vi "PXI_Host_U16_Write_OldMethod_Benchmark.vi"() -> ()   [LabVIEW 2018]
uses:
  <vilib>/Platform/TimedLoop/XDataNode/timing_clust.ctl
  <vilib>/Platform/TimedLoop/XDataNode/nitl_modes.ctl
  <vilib>/Platform/TimedLoop/XDataNode/wakeup.ctl
  <vilib>/NI/LVFPGA Adv Session Resources/OpenByNameSubVI.vi
  <vilib>/rvi/interface/common/dynamic/niFpgaEscapeDelimiterAndNull.vi
  <vilib>/Utility/error.llb/Error Cluster From Error Code.vi
  <vilib>/rvi/errors/niLvFpgaAdjustHostInterfaceError.vi
  <vilib>/FPGAPlugInAG/Dynamic/niLvFpga_Close_Dynamic.vi
  <vilib>/platform/TimedLoop/XDataNode/XDataNode.xnode
  <vilib>/NI/LVFPGA Adv Session Resources/OpenByName.xnode
  <vilib>/rvi/interface/nirviReadWriteControl/nirviReadWriteControl.xnode
  <vilib>/rvi/interface/nirviCloseFPGA/nirviCloseFPGA.xnode
  NiFpgaLv.dll
  <vilib>/rvi/interface/Simulation/niFpgaSimulationCallBeginRW.vi
  <vilib>/NI/LVFPGA Adv Session Resources/LVFPGAAdvSessionResources.lvlib
  cRIO RT/FPGA Bitfile Register Operations/Scalar IO Operations/FPGA Register IO.lvlib
  <vilib>/Platform/TimedLoop/XDataNode/XDNodeRunTimeDep.lvlib
panel:
  out "Maximum(s)":dbl
  out "Standard deviation":dbl
  out "Waveform Graph":dbl[](graph)
  out "error out":errorcluster
  out "Execution time (s)":dbl
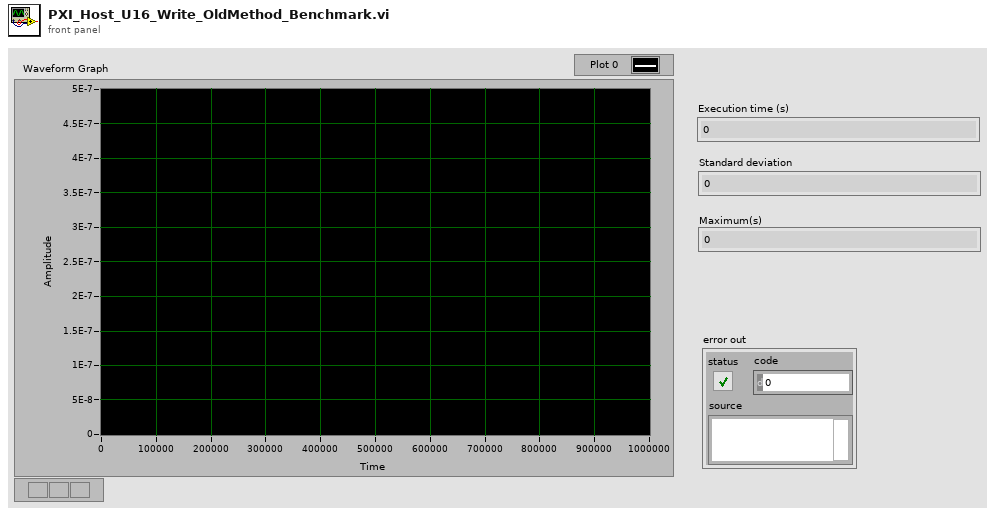
[diagram p1: front panel]
types:
  T1 = typedef "XDNodeRunTimeDep.lvlib/timing_clust.ctl" = cluster{"Expected End [f-1]":u64, "Actual End [f-1]":u64, "Finished Late? [f-1]":bool, "Expected End [i-1]":u64, "Actual End [i-1]":u64, "Finished Late? [i-1]":bool, "Expected Start [i]":u64, "Actual Start [i]":u64, "Expected Start [f]":u64, "Actual Start [f]":u64, "Source Name":string, "Structure Name":string, "Period":i64, "Deadline":i64, "Offset":i64, "Start":i64, "Priority":i32, "Timeout":i32, "Mode":T2, "Wakeup Reason":T3, "Error":errorcluster, "Source Type":string, "Secondary Source Type":string, "Global End Time":u64, "Global Start Time":u64, "Frame Duration":u64, "Iteration Duration":u64, "Assigned CPU":i32, "I/O Scan Engine Mode":u32}
  T2 = typedef "XDNodeRunTimeDep.lvlib/nitl_modes.ctl" = enum32{"No Change", "Process missed periods, maintain original phase", "Discard missed periods, maintain original phase", "Process missed periods, ignore original phase", "Discard missed periods, ignore original phase"}
  T3 = typedef "XDNodeRunTimeDep.lvlib/wakeup.ctl" = enum32{"Normal", "Aborted", "Asynchronous wakeup", "Timing source error", "Timed loop error", "Timeout"}
  T4 = cluster{"Name":string, "Depth":u32, "Write? (Deprecated:Use Implementation)":bool, "Physical Channel":u32, "Base Address":u32, "Data Width":u32, "Data Type":enum32{"Boolean", "I8", "I16", "I32", "I64", "U8", "U16", "U32", "U64", "FXP", "CustomControl", "SGL"}, "FXP Properties":variant, "Write Window Address":u32, "Implementation":enum16{"niFpgaTargetToHost", "niFpgaHostToTarget", "niFpgaPeerToPeerWriter", "niFpgaPeerToPeerReader", "niCoreTargetToHost", "niCoreHostToTarget"}, "Control Set":u32}[]
  T5 = cluster{"Name":string, "type":variant, "indicator?":bool}[]
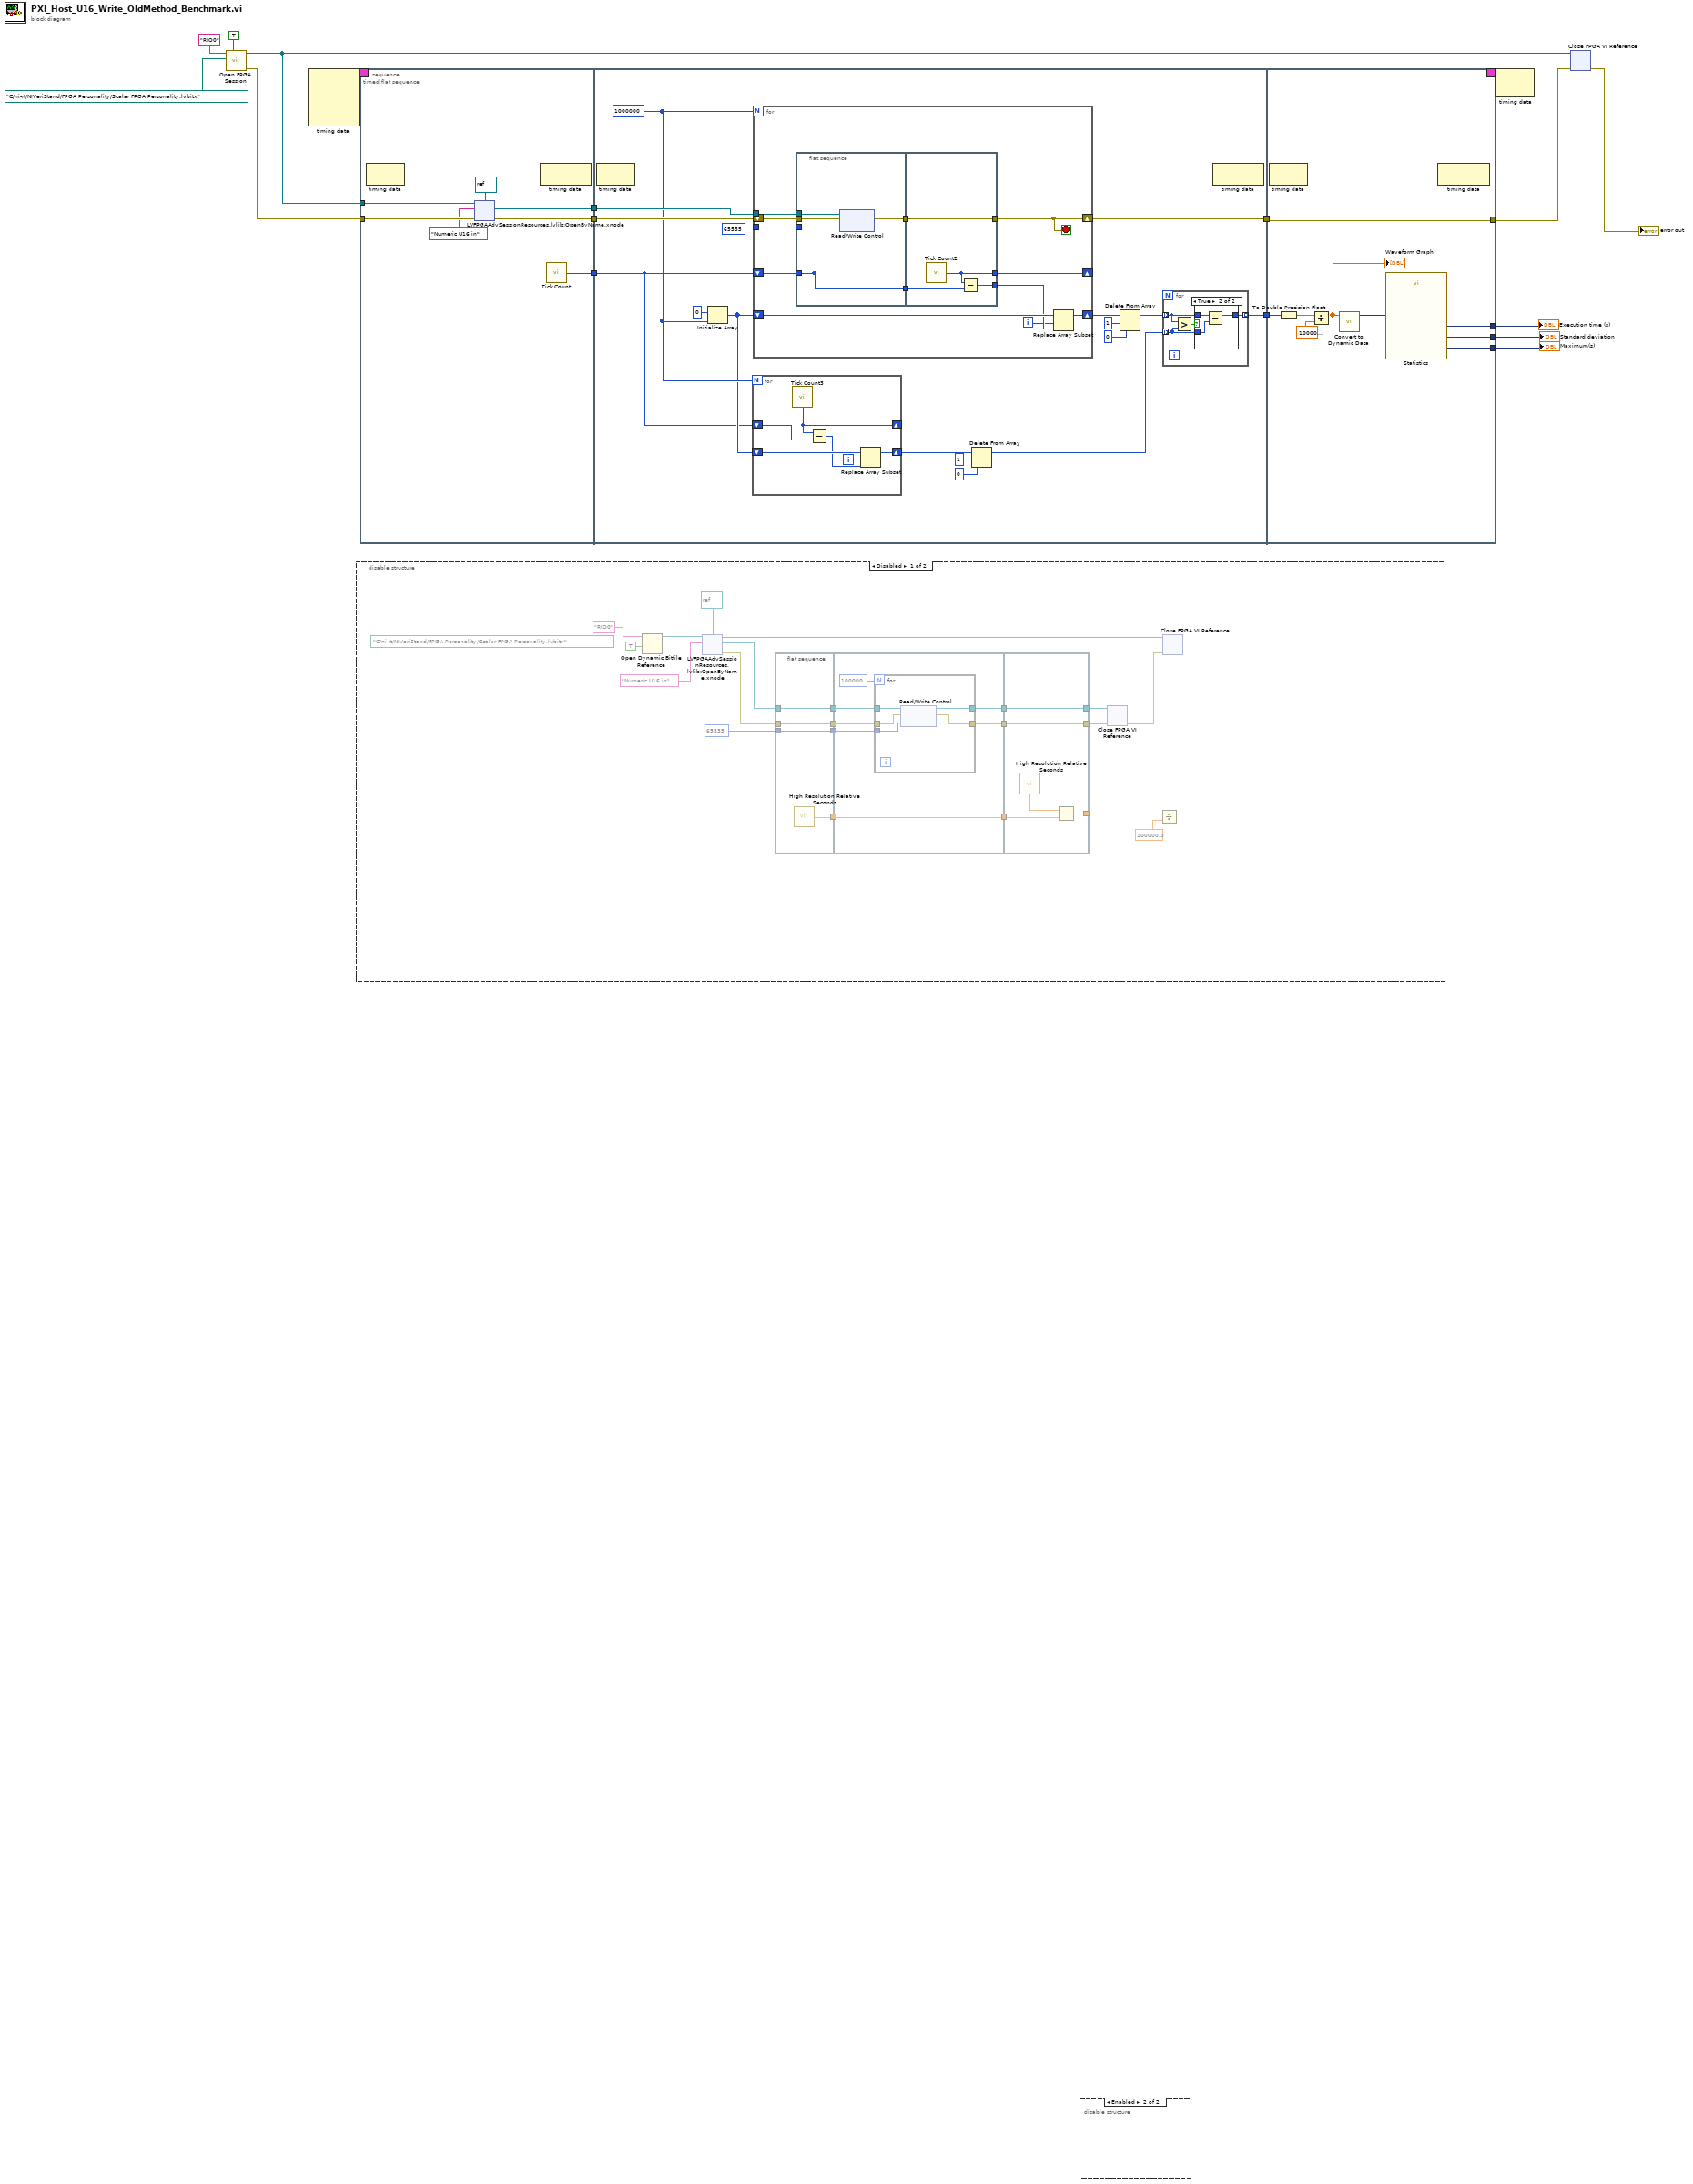
[diagram p0: block diagram]
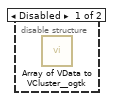
[diagram p4: hidden frame]
diagram:
  n1 = call "Open FPGA Session.vi"("run when loaded (T)"=TRUE, "bitfile path"=path "C:/ni-rt/NIVeriStand/FPGA Personality/Scalar FPGA Personality.lvbitx", "device address"="RIO0") -> ("error out"=w7:errorcluster, "bitfile reference out"=w1:refnum<k20>)  [unwired: 6 in, 1 out]
  n2 = node-c288() -> (w12:T1)  [unwired: 4 in]
  n3 = disable-structure shown="Disabled" {
    frame Disabled {
      n4 = Open Dynamic Bitfile Reference(0:"RIO0" ("Device address"), 1:path "C:/ni-rt/NIVeriStand/FPGA Personality/Scalar FPGA Personality.lvbitx" ("Bitfile path"), 2:TRUE ("Run When Loaded")) -> (5:w22:refnum<k20>, 8:w20:errorcluster)  [unwired: 2 in]
      n5 = xnode "LVFPGAAdvSessionResources.lvlib:OpenByName.xnode"("FPGA VI Reference in"=w22, "Resource name in"="Numeric U16 in", "Single resource reference type in"=refnum<k20> refnum ("Type"), "Error in"=w20) -> ("Single resource reference out"=w18:refnum<k20>, "Error out"=w19:errorcluster, "FPGA VI Reference out"=w14:refnum<k20>)
      n6 = flat-sequence {
        tunnel: [w39] -> w35
        tunnel: w18 -> [w38]
        tunnel: [w38] -> w34
        tunnel: [w37] -> w33
        tunnel: w19 -> [w37]
        tunnel: [w36] -> w32
        tunnel: u16 65535 ("Value") -> [w36]
        tunnel: [w45] -> w31
        tunnel: w35 -> [w45]
        tunnel: w34 -> [w44]
        tunnel: w33 -> [w43]
        tunnel: [w42] -> w30
        tunnel: [w41] -> w29
        tunnel: w32 -> [w40]
        tunnel: w31 -> [w55]
        tunnel: [w54] -> w28
        tunnel: w30 -> [w53]
        tunnel: [w53] -> w23
        tunnel: w29 -> [w52]
        tunnel: [w52] -> w16
        frame #0 {
          n7 = call <vilib>:"High Resolution Relative Seconds.vi"() -> ("relative seconds"=w39:dbl)
        }
        frame #1 {
          n8 = for {
            N: 100000 -> [_]
            tunnel: w44 -> [w51]
            tunnel: w43 -> [w50]
            tunnel: [w49] -> w42
            tunnel: [w48] -> w41
            tunnel: w40 -> [w47]
            n9 = xnode "Read/Write Control"("FPGA VI Reference In"=w51, "error in"=w50, "Value"=w47) -> ("FPGA VI Reference Out"=w48:refnum<k20>, "error out"=w49:errorcluster)
          }
        }
        frame #2 {
          n10 = call <vilib>:"High Resolution Relative Seconds.vi"() -> ("relative seconds"=w56:dbl)
          n11 = Subtract(x=w56, y=w55) -> (x-y=w54:dbl)
        }
      }
      n12 = xnode "Close FPGA VI Reference"("FPGA VI Reference In"=w16, "error in"=w23) -> ("error out"=w15:errorcluster)
      n13 = Divide(x=w28, y=100000.0) -> ()  [unwired: 1 out]
      n14 = xnode "Close FPGA VI Reference"("FPGA VI Reference In"=w14, "error in"=w15) -> ()  [unwired: 1 out]
    }
    frame Enabled {
    }
  }
  n15 = timed-sequence {
    timing: w12 -> [_]
    timing-out: [_] -> w11
    tunnel: w7 -> [w72]
    tunnel: [w77] -> w6
    tunnel: [w75] -> w4
    tunnel: [w74] -> w3
    tunnel: [w73] -> w2
    tunnel: w1 -> [w71]
    n16 = timed-flat-sequence {
      tunnel: [w84] -> w80
      tunnel: [w85] -> w79
      tunnel: [w87] -> w76
      tunnel: w72 -> [w83]
      tunnel: w71 -> [w86]
      tunnel: w80 -> [w119]
      tunnel: [w118] -> w78
      tunnel: w79 -> [w117]
      tunnel: w76 -> [w107]
      tunnel: [w103] -> w70
      tunnel: w78 -> [w165]
      tunnel: [w165] -> w77
      tunnel: [w163] -> w75
      tunnel: [w160] -> w74
      tunnel: [w159] -> w73
      tunnel: w70 -> [w158]
      frame #0 {
        n17 = node-c288() -> ()  [unwired: 1 in, 1 out]
        n18 = xnode "LVFPGAAdvSessionResources.lvlib:OpenByName.xnode"("FPGA VI Reference in"=w86, "Resource name in"="Numeric U16 in", "Single resource reference type in"=refnum<k20> refnum ("Type"), "Error in"=w83) -> ("Single resource reference out"=w85:refnum<k20>, "Error out"=w84:errorcluster)  [unwired: 1 out]
        n19 = node-c288() -> ()  [unwired: 1 in, 1 out]
        n20 = call "Tick Count"() -> ("Tick Count(Ticks)"=w87:u32)
      }
      frame #1 {
        w109 = 1000000
        n21 = node-c288() -> ()  [unwired: 1 in, 1 out]
        n22 = Initialize Array(u32 0, w109) -> (w108:u32[])
        n23 = for {
          N: w109 -> [_]
          shift-right: [w128] -> w110
          shift-left: w108 -> [w131]
          shift-right: [w133] -> _
          shift-left: w107 -> [w132]
          i -> [w129]
          n24 = call "Tick Count3"() -> ("Tick Count(Ticks)"=w133:u32)
          n25 = Subtract(x=w133, y=w132) -> (x-y=w130:u32)
          n26 = Replace Array Subset(array=w131, new element=w130, index=w129) -> (w128:u32[])
        }
        n27 = for {
          N: w109 -> [_]
          tunnel: w117 -> [w146]
          shift-right: [w144] -> _
          shift-left: w107 -> [w143]
          shift-right: [w139] -> w115
          shift-left: w108 -> [w141]
          shift-right: [w137] -> w118
          shift-left: w119 -> [w147]
          tunnel: u16 65535 ("Value") -> [w136]
          i -> [w138]
          stop <- w137 stop-if-true
          n28 = flat-sequence {
            tunnel: w147 -> [w151]
            tunnel: w146 -> [w149]
            tunnel: [w150] -> w145
            tunnel: [w152] -> _
            tunnel: w143 -> [w152]
            tunnel: [w152] -> w142
            tunnel: w136 -> [w148]
            tunnel: [w156] -> w137
            tunnel: w145 -> [w156]
            tunnel: [w155] -> w144
            tunnel: w142 -> [w154]
            tunnel: [w153] -> w140
            frame #0 {
              n29 = xnode "Read/Write Control"("FPGA VI Reference In"=w149, "error in"=w151, "Value"=w148) -> ("error out"=w150:errorcluster)  [unwired: 1 out]
            }
            frame #1 {
              n30 = call "Tick Count2"() -> ("Tick Count(Ticks)"=w155:u32)
              n31 = Subtract(x=w155, y=w154) -> (x-y=w153:u32)
            }
          }
          n32 = Replace Array Subset(array=w141, new element=w140, index=w138) -> (w139:u32[])
        }
        n33 = Delete From Array(array=w110, length=1, index=0) -> (array with subset deleted=w104:u32[])  [unwired: 1 out]
        n34 = Delete From Array(array=w115, length=1, index=0) -> (array with subset deleted=w105:u32[])  [unwired: 1 out]
        n35 = for {
          tunnel: [w123] -> w103 mode=indexing
          tunnel: w105 -> [w122] mode=indexing
          tunnel: w104 -> [w121] mode=indexing
          n36 = Greater?(x=w122, y=w121) -> (0:w120:bool)
          n37 = case shown="True" w120 {
            tunnel: w122 -> [w124 w127]
            tunnel: w121 -> [_ w126]
            tunnel: [w124 w125] -> w123
            frame False {
            }
            frame True {
              n38 = Subtract(x=w127, y=w126) -> (x-y=w125:u32)
            }
          }
        }
        n39 = node-c288() -> ()  [unwired: 1 in, 1 out]
      }
      frame #2 {
        n40 = node-c288() -> ()  [unwired: 1 in, 1 out]
        n41 = To Double Precision Float(number=w158) -> (double precision float=w162:dbl[])
        n42 = Divide(x=w162, y=1000000000.0) -> (x/y=w157:dbl[])
        "Waveform Graph" <- w157
        n43 = call "Convert to Dynamic Data"("Array"=w157) -> ("Dynamic Data Type"=w164:dynamicdata)  [unwired: 3 in]
        n44 = call "Statistics"("Signals"=w164) -> ("Standard Dev"=w160:dynamicdata, "Arithmetic Mean"=w163:dynamicdata, "Maximum"=w159:dynamicdata)  [unwired: 23 in, 1 out]
        n45 = node-c288() -> ()  [unwired: 1 in, 1 out]
      }
    }
  }
  "Execution time (s)" <- w4
  "Standard deviation" <- w3
  "Maximum(s)" <- w2
  n46 = disable-structure shown="Enabled" {
    frame Disabled {
      n47 = call <userlib>:"Array of VData to VCluster__ogtk.vi"() -> ()  [unwired: 10 in, 2 out]
    }
    frame Enabled {
    }
  }
  n48 = node-c288(w11) -> ()  [unwired: 1 out]
  n49 = xnode "Close FPGA VI Reference"("FPGA VI Reference In"=w1, "error in"=w6) -> ("error out"=→"error out":errorcluster)
